vi "MDP_BMS_DTC.vi"(8 "errin":errorcluster, 9 "Channel out":T1, 10 "SA":u32=64 format="%.0x", 11 "TA":u32 format="%.0x") -> (0 "errout":errorcluster, 3 "OK":bool)   [LabVIEW 2020]
uses:
  C/Program Files (x86)/National Instruments/LabVIEW 2020/user.lib/PCAN Basic/Controls/Channel.ctl
  C/Program Files (x86)/National Instruments/LabVIEW 2020/user.lib/Alex_Peak_lib/PEAK_lib_ALEX.lvlib
  C/Program Files (x86)/National Instruments/LabVIEW 2020/user.lib/PCAN Basic/PCANBasic.lvlib
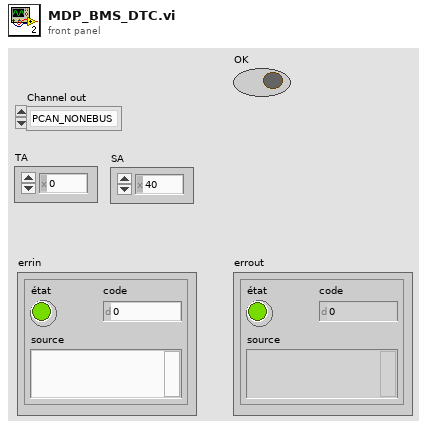
[diagram p1: front panel]
types:
  T1 = typedef "PCANBasic.lvlib/Channel.ctl" = enum16{"PCAN_NONEBUS", "not used1", "not used2", "not used3", "not used4", "not used5", "not used6", "not used7", "not used8", "not used9", "not used10", "not used11", "not used12", "not used13", "not used14", "not used15", "not used16", "not used17", "not used18", "not used19", "not used20", "not used21", "not used22", "not used23", "not used24", "not used25", "not used26", "not used27", "not used28", "not used29", "not used30", "not used31", "not used32", "PCAN_ISABUS1", "PCAN_ISABUS2", "PCAN_ISABUS3", "PCAN_ISABUS4", "PCAN_ISABUS5", "PCAN_ISABUS6", "PCAN_ISABUS7", "PCAN_ISABUS8", "not used41", "not used42", "not used43", "not used44", "not used45", "not used46", "not used47", "not used48", "PCAN_DNGBUS1", "not used50", "not used51", "not used52", "not used53", "not used54", "not used55", "not used56", "not used57", "not used58", "not used59", "not used60", "not used61", "not used62", "not used63", "not used64", "PCAN_PCIBUS1", "PCAN_PCIBUS2", "PCAN_PCIBUS3", "PCAN_PCIBUS4", "PCAN_PCIBUS5", "PCAN_PCIBUS6", "PCAN_PCIBUS7", "PCAN_PCIBUS8", "not used73", "not used74", "not used75", "not used76", "not used77", "not used78", "not used79", "not used80", "PCAN_USBBUS1", "PCAN_USBBUS2", "PCAN_USBBUS3", "PCAN_USBBUS4", "PCAN_USBBUS5", "PCAN_USBBUS6", "PCAN_USBBUS7", "PCAN_USBBUS8", "Not used89", "Not used90", "Not used91", "Not used92", "Not used93", "Not used94", "Not used95", "Not used96", "PCAN_PCCBUS1", "PCAN_PCCBUS2"}
  T2 = cluster{"ID":u32, "MSGTYPE":u8, "LEN":u8, "DATA[0]":u8, "DATA[1]":u8, "DATA[2]":u8, "DATA[3]":u8, "DATA[4]":u8, "DATA[5]":u8, "DATA[6]":u8, "DATA[7]":u8}
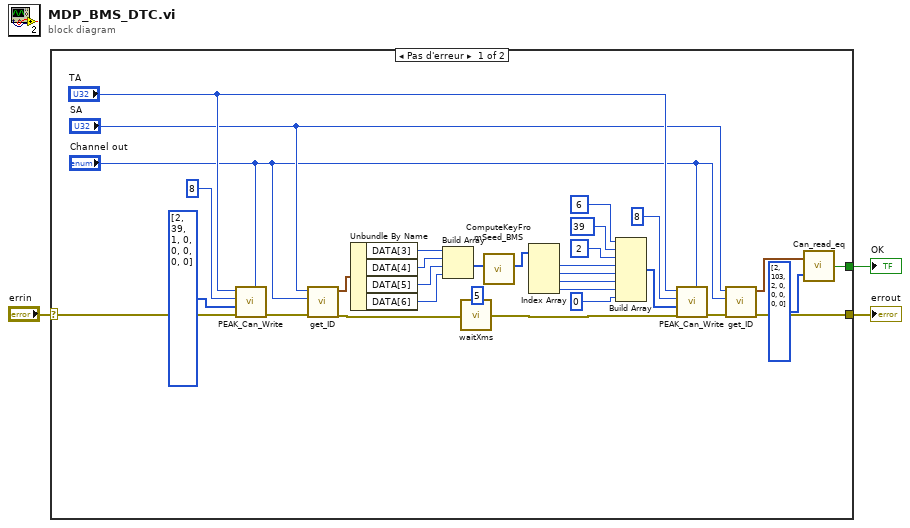
[diagram p0: block diagram]
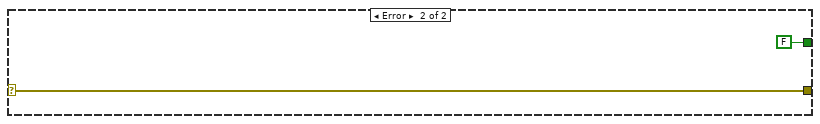
[diagram p2: hidden frame]
diagram:
  n1 = case shown="Pas d'erreur" "errin" {
    selector: "errin" -> [w12 w36]
    tunnel: [w31 w36] -> w3
    tunnel: [w11 FALSE ("Identique")] -> w1
    frame No Error {
      (unwired) u32 5 ("attente (ms)")
      n2 = call "PEAK_Can_Write.vi"("CAN Handle"="Channel out", "errin"=w12, "CAN Data"=u8[] [2, 39, 1, 0, 0, 0, 0, 0], "DLC (8)"=u8 8, "Identifier"="TA") -> ("errout"=w15:errorcluster)  [unwired: 6 in]
      n3 = call "get_ID.vi"("errin"=w15, "ChannelIn"="Channel out", "Identifier"="SA") -> ("errout"=w10:errorcluster, "Messout"=w29:T2)  [unwired: 5 in, 2 out]
      n4 = Unbundle By Name(w29) -> ("DATA[3]"=w16:u8, "DATA[4]"=w19:u8, "DATA[5]"=w18:u8, "DATA[6]"=w17:u8)
      n5 = Build Array(w16, w19, w18, w17) -> (w6:u8[])
      n6 = call "waitXms.vi"("errin"=w10) -> ("errout"=w9:errorcluster)  [unwired: 14 in]
      n7 = call "ComputeKeyFromSeed_BMS.vi"("Seed"=w6) -> ("Key"=w5:u8[])  [unwired: 10 in]
      n8 = Index Array(array=w5) -> (element #1=w23:u8, element #2=w24:u8, element #3=w25:u8, element #4=w26:u8)  [unwired: 4 in]
      n9 = Build Array(u32 6 ("Identifier"), u32 39 ("Identifier"), u32 2 ("Identifier"), w23, w24, w25, w26, u32 0 ("élément")) -> (w27:u32[])
      n10 = call "PEAK_Can_Write.vi"("CAN Handle"="Channel out", "errin"=w9, "CAN Data"=w27, "DLC (8)"=u8 8, "Identifier"="TA") -> ("errout"=w32:errorcluster)  [unwired: 6 in]
      n11 = call "get_ID.vi"("errin"=w32, "ChannelIn"="Channel out", "Identifier"="SA") -> ("errout"=w31:errorcluster, "Messout"=w33:T2)  [unwired: 5 in, 2 out]
      n12 = call "Can_read_eq.vi"("TrameJeVeux"=u8[] [2, 103, 2, 0, 0, 0, 0, 0], "MessIN"=w33) -> ("Identique"=w11:bool)
    }
    frame Error {
    }
  }
  "errout" <- w3
  "OK" <- w1
